vi "Handle Type Name.vi"(8 "error in (no error)":errorcluster, 9 "Type":refnum<class>, 10 "JSON":string, 11 "Flatten To JSON Object in":refnum<class "Flatten To JSON Object.lvclass">) -> (0 "error out":errorcluster, 1 "Type out":refnum<class>, 2 "JSON out":string, 3 "Flatten To JSON Object out":refnum<class "Flatten To JSON Object.lvclass">)   [LabVIEW 2017, in "Flatten To JSON Object.lvclass"]
doc: "Extracts type information from a JSON object."
uses:
  Flatten To JSON Object.lvclass
  Flatten To JSON Object.lvclass/Flatten To JSON Object.ctl
  Serialization Binder/Serialization Binder.lvclass
  <vilib>/JDP Science/JSONtext/JSONtext.lvlib
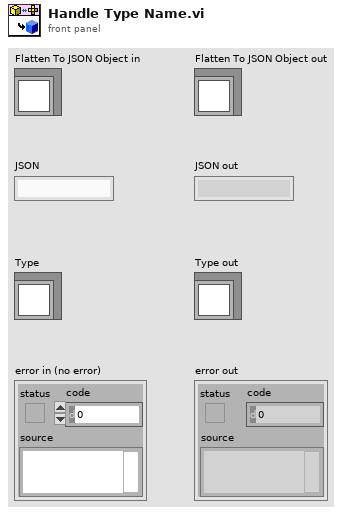
[diagram p1: front panel]
types:
  T1 = typedef "Flatten To JSON Object.lvclass/Type Name Handling.ctl" = enum16{"None", "Inline"}
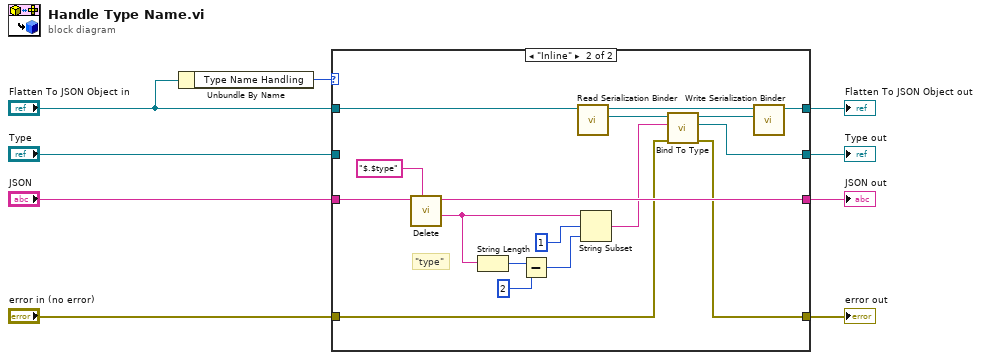
[diagram p0: block diagram]
diagram:
  n1 = Unbundle By Name("Flatten To JSON Object in") -> ("Type Name Handling"=w7:T1)
  n2 = case shown="\"Inline\"" w7 {
    tunnel: "Flatten To JSON Object in" -> [w13 w18]
    tunnel: [w13 w16] -> w8
    tunnel: "JSON" -> [w12 w21]
    tunnel: [w12 w29] -> w5
    tunnel: [w11 w24] -> w4
    tunnel: "Type" -> [w11 _]
    tunnel: "error in (no error)" -> [w10 w20]
    tunnel: [w10 w19] -> w1
    frame Default {
    }
    frame "Inline" {
      # "\"type\""
      n3 = call <vilib>:"Delete.vi"("$Path or Item Name"="$.$type", "JSON"=w21) -> ("<JSON> First Deleted Item"=w22:string, "<JSON>"=w29:string)  [unwired: 5 in, 2 out]
      n4 = String Length(string=w22) -> (length=w27:i32)
      n5 = Subtract(x=w27, y=2) -> (x-y=w25:i32)
      n6 = call "Read Serialization Binder.vi"("Flatten To JSON Object in"=w18) -> ("Serialization Binder"=w15:refnum<class "Serialization Binder.lvclass">, "Flatten To JSON Object out"=w17:refnum<class "Flatten To JSON Object.lvclass">)  [unwired: 8 in, 1 out]
      n7 = String Subset(string=w22, offset (0)=1, length (rest)=w25) -> (substring=w23:string)
      n8 = call-dynamic "Bind To Type.vi"("error in (no error)"=w20, "Type Name"=w23, "Serialization Binder in"=w15) -> ("error out"=w19:errorcluster, "Type"=w24:refnum<class>, "Serialization Binder out"=w14:refnum<class "Serialization Binder.lvclass">)  [unwired: 6 in]
      n9 = call "Write Serialization Binder.vi"("Serialization Binder"=w14, "Flatten To JSON Object in"=w17) -> ("Flatten To JSON Object out"=w16:refnum<class "Flatten To JSON Object.lvclass">)  [unwired: 8 in, 1 out]
    }
  }
  "error out" <- w1
  "Flatten To JSON Object out" <- w8
  "JSON out" <- w5
  "Type out" <- w4
